vi "niRFUtil FWK Match Whole Word.vi"(8 "error in":errorcluster, 9 "Search String":string, 10 "Input String":string) -> (0 "error out":errorcluster, 2 "Whole Word Matched?":bool)   [LabVIEW 2015, in "niRFUtil.lvlib"]
uses:
  niRFUtil.lvlib
  <vilib>/regexp/Match Regular Expression.xnode
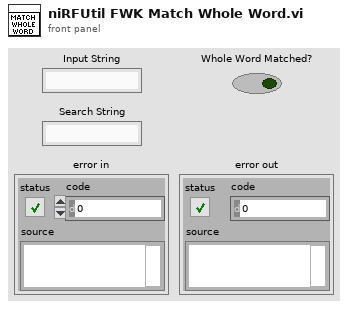
[diagram p1: front panel]
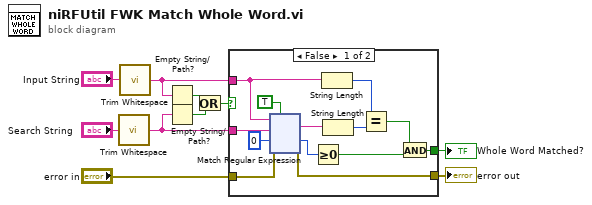
[diagram p0: block diagram]
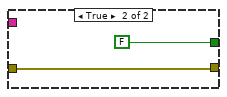
[diagram p2: hidden frame]
diagram:
  n1 = call <vilib>:"Trim Whitespace.vi"("string"="Search String") -> ("trimmed string"=w5:string)  [unwired: 1 in]
  n2 = call <vilib>:"Trim Whitespace.vi"("string"="Input String") -> ("trimmed string"=w4:string)  [unwired: 1 in]
  n3 = Empty String/Path?(string/path=w4) -> (empty?=w3:bool)
  n4 = Empty String/Path?(string/path=w5) -> (empty?=w2:bool)
  n5 = Or(x=w3, y=w2) -> (x .or. y?=w1:bool)
  n6 = case shown="False" w1 {
    tunnel: [w23 FALSE] -> w10
    tunnel: w4 -> [w17 _]
    tunnel: "error in" -> [w14 w139]
    tunnel: [w13 w139] -> w6
    tunnel: w5 -> [w11 _]
    frame False {
      n7 = xnode "Match Regular Expression"("input string"=w17, "regular expression"=w11, "offset (0)"=0, "error in"=w14, "ignore case? (F)"=TRUE) -> ("whole match"=w16:string, "offset past match"=w20:i32, "error out"=w13:errorcluster)  [unwired: 1 in, 2 out]
      n8 = Greater Or Equal To 0?(x=w20) -> (x >= 0?=w22:bool)
      n9 = String Length(string=w17) -> (length=w19:i32)
      n10 = String Length(string=w16) -> (length=w18:i32)
      n11 = Equal?(x=w19, y=w18) -> (x = y?=w21:bool)
      n12 = And(x=w21, y=w22) -> (x .and. y?=w23:bool)
    }
    frame True {
    }
  }
  "Whole Word Matched?" <- w10
  "error out" <- w6
